vi "VNA_close_if_error.vi"(8 "error in (no error)":errorcluster, 11 "IVI Refnum in":refnum<k15>) -> (0 "error out":errorcluster, 3 "IVI Refnum out":refnum<k15>)   [LabVIEW 2016]
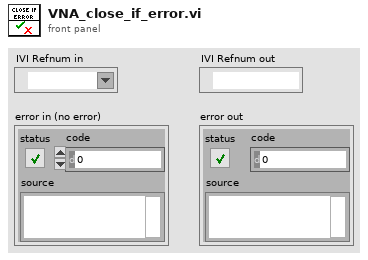
[diagram p1: front panel]
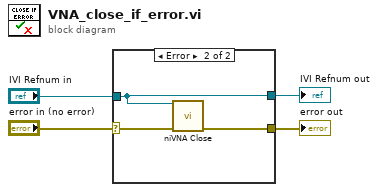
[diagram p0: block diagram]
diagram:
  n1 = case shown="Error" "error in (no error)" {
    selector: "error in (no error)" -> [w5 w9]
    tunnel: [w6 w7] -> w1
    tunnel: "IVI Refnum in" -> [w6 w7]
    tunnel: [w5 w8] -> w3
    frame No Error {
    }
    frame Error {
      n2 = call <instrlib>:"niVNA Close.vi"("instrument handle"=w7, "error in"=w9) -> ("error out"=w8:errorcluster)  [unwired: 13 in]
    }
  }
  "error out" <- w3
  "IVI Refnum out" <- w1
